vi "Spectrometer Controller.vi"(8 "error in (no error)":errorcluster, 10 "Notifiers":T1, 11 "All Message Queue Cluster":T2) -> (0 "error out":errorcluster)   [LabVIEW 2017]
uses:
  Lib QMH/AllMessageQueue Cluster.ctl
  Lib QMH/Message Cluster.ctl
  Lib Notifier/Notifier.ctl
  Lib Log/Logging.lvlib
  Lib QMH/MessageQueues.lvlib
  Lib Notifier/Notifier.lvlib
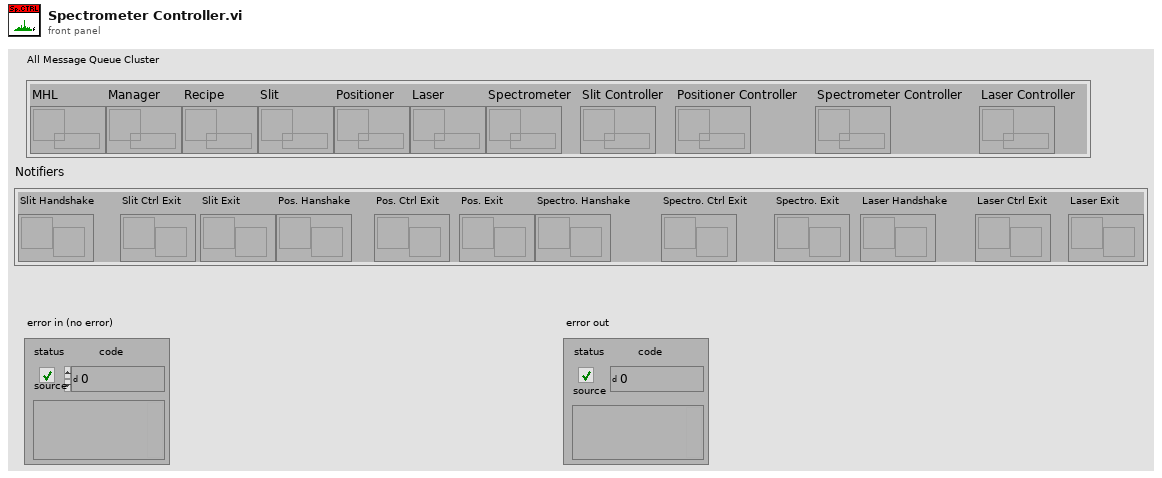
[diagram p1: front panel]
types:
  T1 = typedef "Notifier.lvlib/Notifier.ctl" = cluster{"Slit Handshake":refnum<notifier>, "Slit Ctrl Exit":refnum<notifier>, "Slit Exit":refnum<notifier>, "Pos. Hanshake":refnum<notifier>, "Pos. Ctrl Exit":refnum<notifier>, "Pos. Exit":refnum<notifier>, "Spectro. Hanshake":refnum<notifier>, "Spectro. Ctrl Exit":refnum<notifier>, "Spectro. Exit":refnum<notifier>, "Laser Handshake":refnum<notifier>, "Laser Ctrl Exit":refnum<notifier>, "Laser Exit":refnum<notifier>}
  T2 = typedef "MessageQueues.lvlib/AllMessageQueue Cluster.ctl" = cluster{"MHL":refnum<queue>, "Manager":refnum<queue>, "Recipe":refnum<queue>, "Slit":refnum<queue>, "Positioner":refnum<queue>, "Laser":refnum<queue>, "Spectrometer":refnum<queue>, "Slit Controller":refnum<queue>, "Positioner Controller":refnum<queue>, "Spectrometer Controller":refnum<queue>, "Laser Controller":refnum<queue>}
  T3 = enum16{"open", "replace", "create", "open or create", "replace or create", "replace or create with confirmation"}
  T4 = cluster{"état":bool, "code":i32, "source":string}
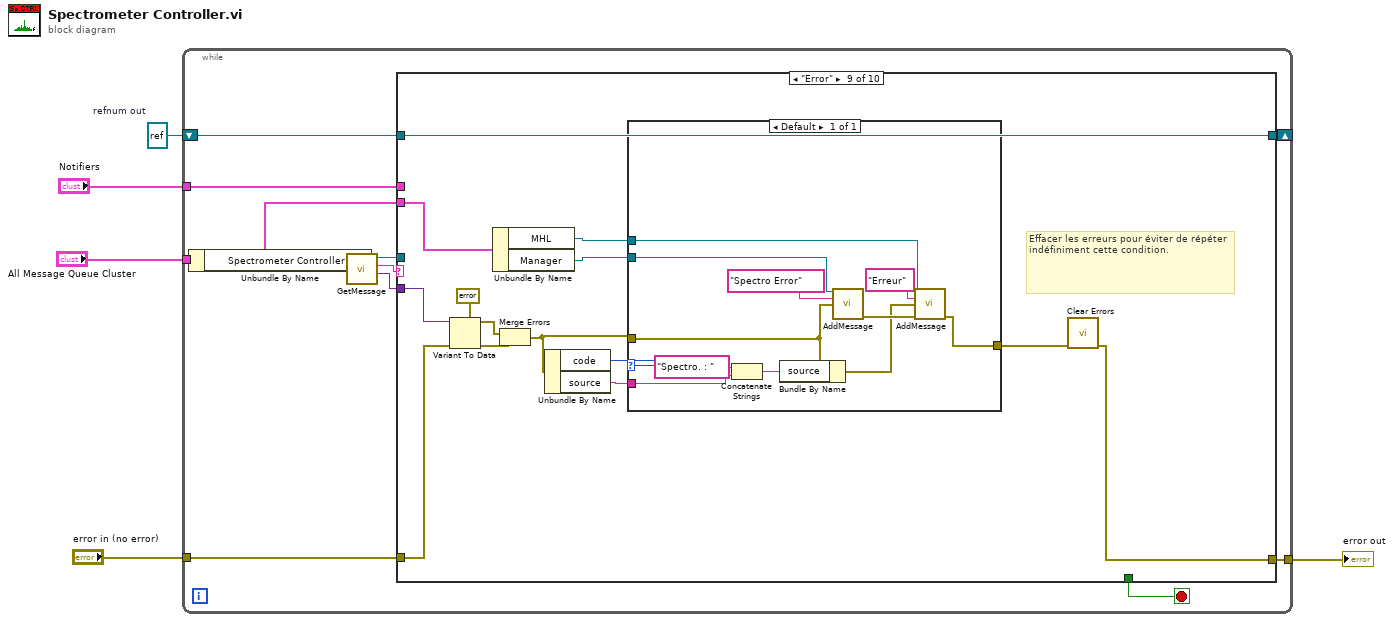
[diagram p0: block diagram]
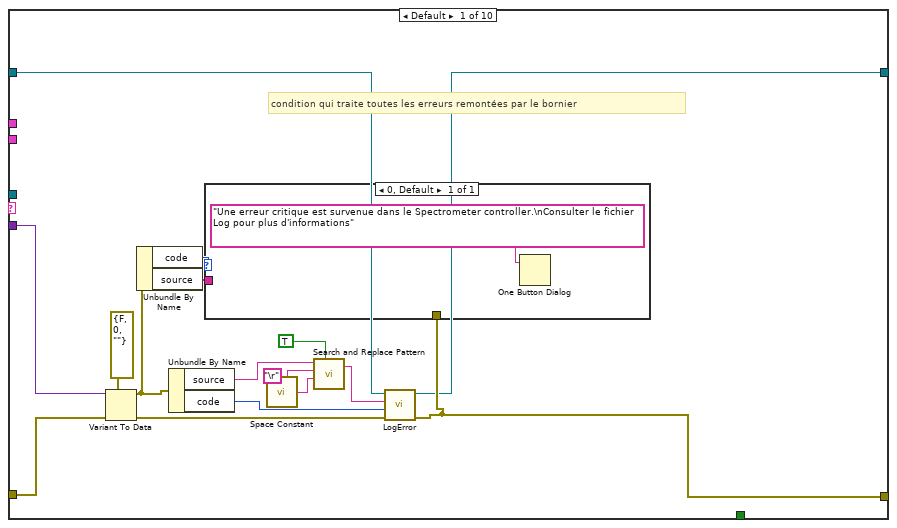
[diagram p2: hidden frame]
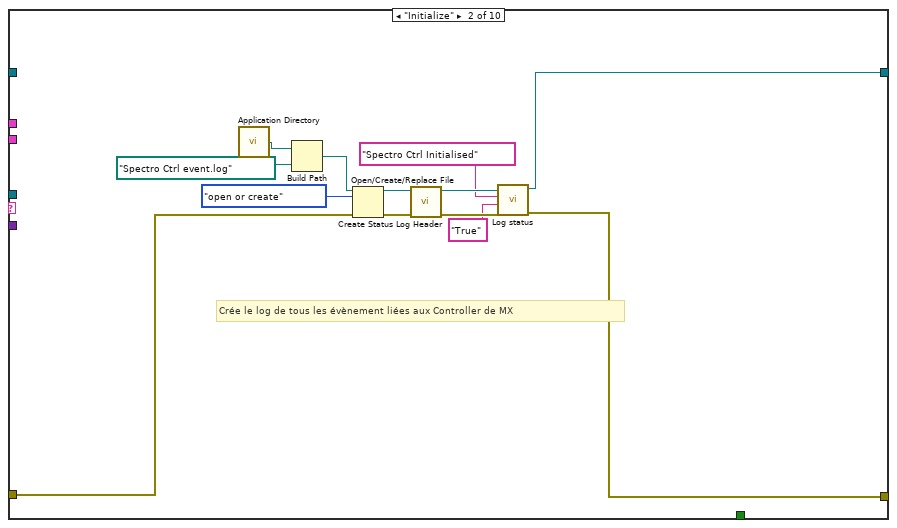
[diagram p3: hidden frame]
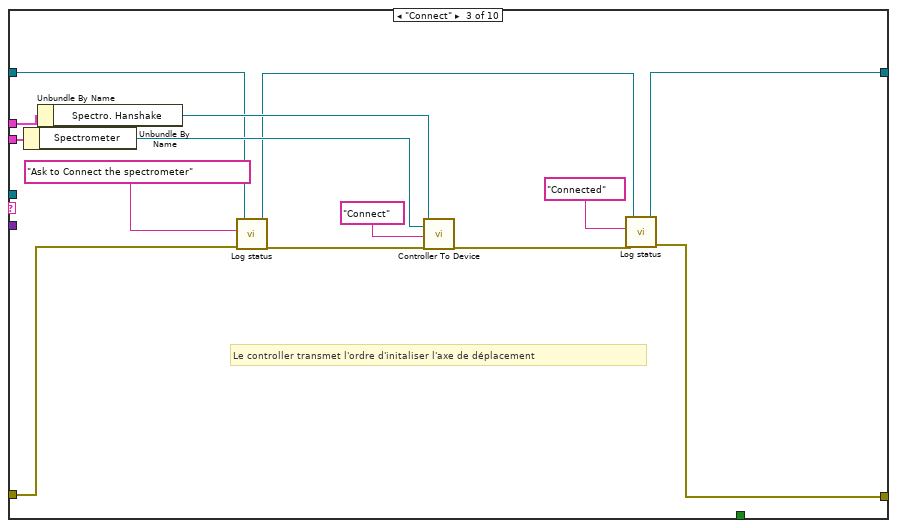
[diagram p4: hidden frame]
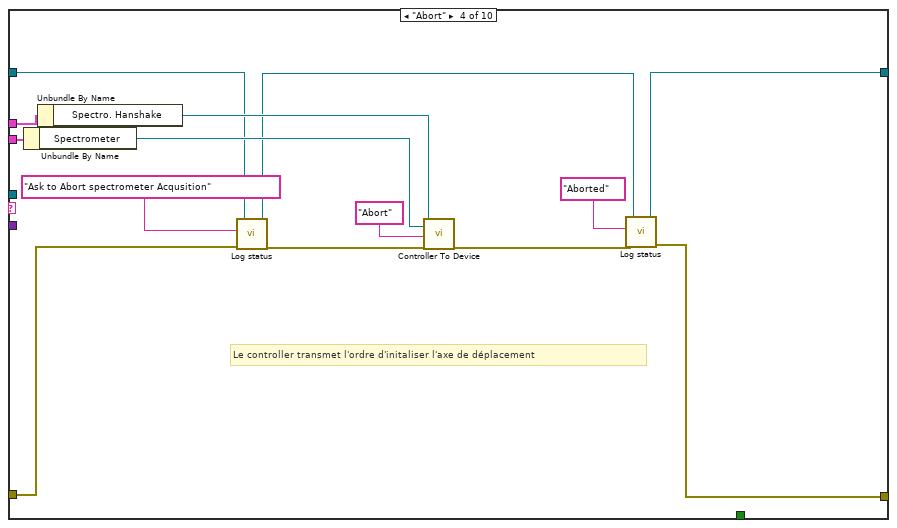
[diagram p5: hidden frame]
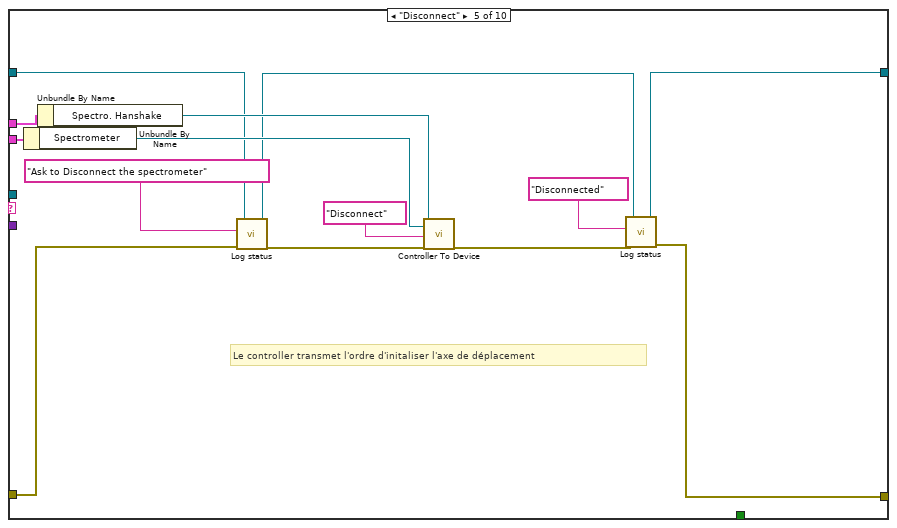
[diagram p6: hidden frame]
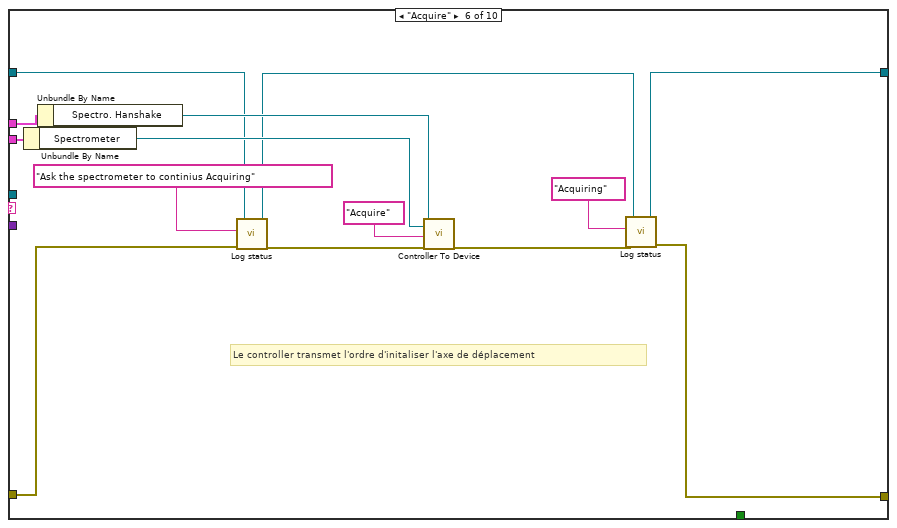
[diagram p7: hidden frame]
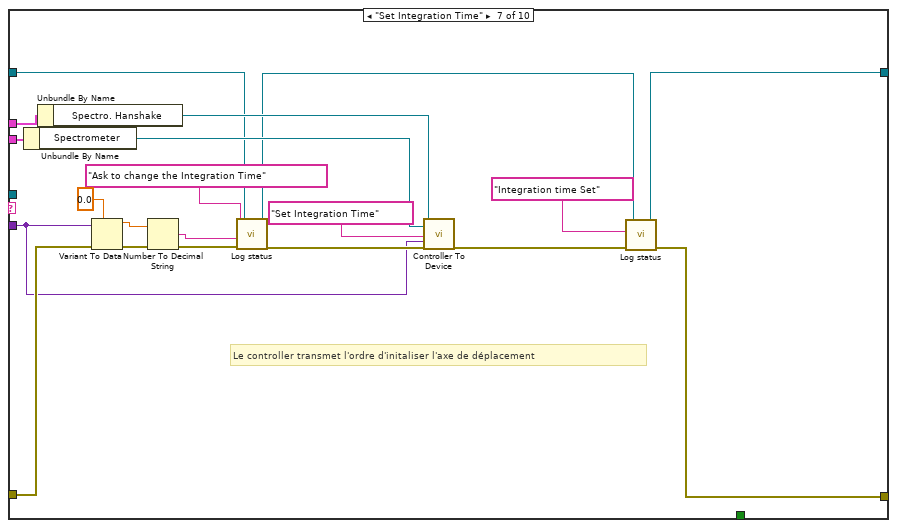
[diagram p8: hidden frame]
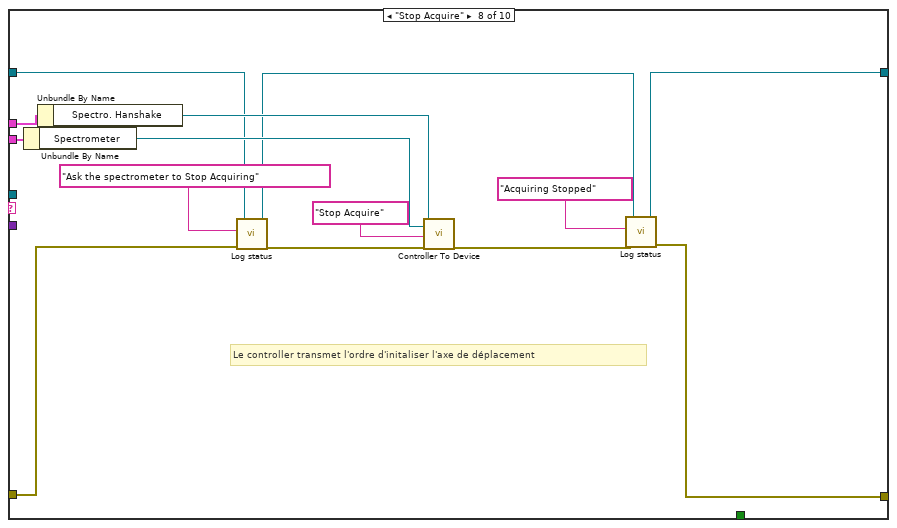
[diagram p9: hidden frame]
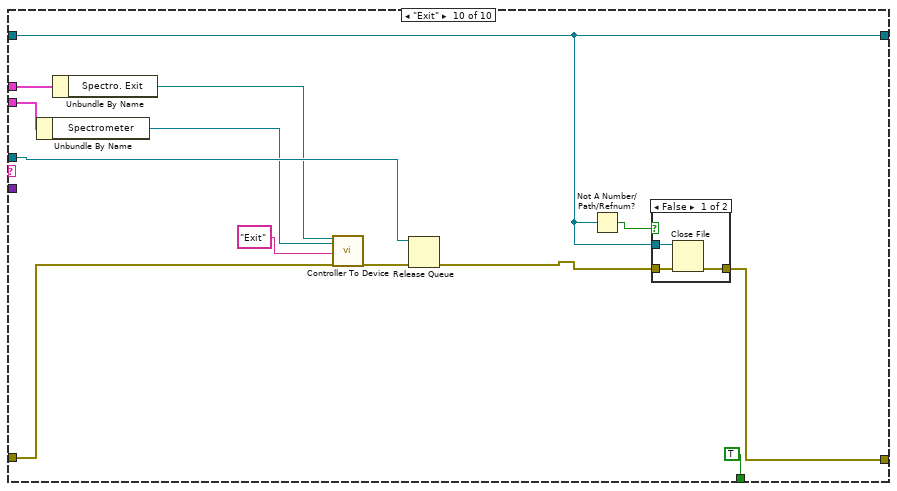
[diagram p10: hidden frame]
diagram:
  w2 = refnum<file> refnum  # refnum out
  n1 = while {
    tunnel: "All Message Queue Cluster" -> [w14]
    tunnel: "Notifiers" -> [w15]
    tunnel: "error in (no error)" -> [w13]
    tunnel: [w6] -> w1
    shift-right: [w8] -> _
    shift-left: w2 -> [w7]
    stop <- w12 stop-if-true
    n2 = Unbundle By Name(w14) -> ("Spectrometer Controller"=w16:refnum<queue>)
    n3 = call "GetMessage.vi"("Message queue"=w16) -> ("Data"=w9:variant, "Message"=w10:string, "Dup Message Queue"=w11:refnum<queue>)  [unwired: 7 in, 1 out]
    n4 = case shown="\"Error\"" w10 {
      tunnel: w15 -> [_ _ w60 w74 w88 w102 w121 w135 _ w170]
      tunnel: w14 -> [_ _ w59 w73 w87 w101 w120 w134 w138 w169]
      tunnel: w13 -> [w21 w36 w48 w62 w76 w90 w108 w123 w140 w165]
      tunnel: [_ _ _ _ _ _ _ _ _ TRUE] -> w12
      tunnel: w11 -> [_ _ _ _ _ _ _ _ _ w171]
      tunnel: w9 -> [w19 _ _ _ _ _ w106 _ w141 _]
      tunnel: [w17 w34 w51 w65 w79 w93 w112 w126 w149 w167] -> w8
      tunnel: w7 -> [w18 _ w55 w69 w83 w97 w116 w130 w149 w167]
      tunnel: [w20 w35 w53 w67 w81 w95 w114 w128 w139 w168] -> w6
      frame Default {
        # "condition qui traite toutes les erreurs remontées par le bornier"
        n5 = Variant To Data(error in=w21, type=errorcluster {"status"=FALSE, "code"=0, "source"=""} ("error in (no error)"), Variant=w19) -> (data=w32:errorcluster, error out=w23:errorcluster)
        n6 = Unbundle By Name(w32) -> ("code"=w30:i32, "source"=w31:string)
        n7 = Unbundle By Name(w32) -> ("source"=w25:string, "code"=w24:i32)
        n8 = call <vilib>:"Space Constant.vi"() -> ("String"=w27:string)
        n9 = call <vilib>:"Search and Replace Pattern.vi"("string"=w25, "regular expression (\"\")"="\r", "replace string (\"\")"=w27, "replace all? (F)"=TRUE) -> ("result string"=w28:string)  [unwired: 1 in, 1 out]
        n10 = call "LogError.vi"("entrée d'erreur"=w23, "Code"=w24, "Source"=w28, "Error log refnum In"=w18) -> ("error out"=w20:errorcluster, "Error log refnum out"=w17:refnum<file>)  [unwired: 6 in]
        n11 = case shown="0, Default" w30 {
          tunnel: w31 -> [_]
          tunnel: w20 -> [_]
          frame 0, Default {
            n12 = One Button Dialog(message="Une erreur critique est survenue dans le Spectrometer controller.\nConsulter le fichier Log pour plus d'informations" ("chaîne de format")) -> ()  [unwired: 1 in, 1 out]
          }
        }
      }
      frame "Initialize" {
        # "Crée le log de tous les évènement liées aux Controller de MX"
        n13 = call <vilib>:"Application Directory.vi"() -> ("Application Directory"=w43:path)
        n14 = Build Path(base path=w43, name or relative path=path "Spectro Ctrl event.log") -> (appended path=w45:path)
        n15 = Open/Create/Replace File(file path (use dialog)=w45, error in=w36, operation (0:open)=T3."open or create" ("opération (0 : open)")) -> (refnum out=w41:refnum<file>, error out=w42:errorcluster)  [unwired: 3 in, 1 out]
        n16 = call "Create Status Log Header.vi"("entrée d'erreur"=w42, "Log File Refnum In"=w41) -> ("sortie d'erreur"=w40:errorcluster, "Log File Refnum out"=w39:refnum<file>)  [unwired: 8 in]
        n17 = call "Log status.vi"("entrée d'erreur"=w40, "Event Data String (-)"="True", "Event string"="Spectro Ctrl Initialised", "Log File Refnum In"=w39) -> ("error out"=w35:errorcluster, "Log File Refnum out"=w34:refnum<file>)  [unwired: 6 in]
      }
      frame "Connect" {
        # "Le controller transmet l'ordre d'initaliser l'axe de déplacement"
        n18 = Unbundle By Name(w59) -> ("Spectrometer"=w57:refnum<queue>)
        n19 = Unbundle By Name(w60) -> ("Spectro. Hanshake"=w58:refnum<notifier>)
        n20 = call "Log status.vi"("entrée d'erreur"=w48, "Event string"="Ask to Connect the spectrometer", "Log File Refnum In"=w55) -> ("error out"=w56:errorcluster, "Log File Refnum out"=w52:refnum<file>)  [unwired: 7 in]
        n21 = call "Controller To Device.vi"("Notifier"=w58, "Message queue"=w57, "Message"="Connect", "entrée d'erreur"=w56) -> ("sortie d'erreur"=w54:errorcluster)  [unwired: 13 in, 2 out]
        n22 = call "Log status.vi"("entrée d'erreur"=w54, "Event string"="Connected", "Log File Refnum In"=w52) -> ("error out"=w53:errorcluster, "Log File Refnum out"=w51:refnum<file>)  [unwired: 7 in]
      }
      frame "Abort" {
        # "Le controller transmet l'ordre d'initaliser l'axe de déplacement"
        n23 = Unbundle By Name(w73) -> ("Spectrometer"=w71:refnum<queue>)
        n24 = Unbundle By Name(w74) -> ("Spectro. Hanshake"=w72:refnum<notifier>)
        n25 = call "Log status.vi"("entrée d'erreur"=w62, "Event string"="Ask to Abort spectrometer Acqusition", "Log File Refnum In"=w69) -> ("error out"=w70:errorcluster, "Log File Refnum out"=w66:refnum<file>)  [unwired: 7 in]
        n26 = call "Controller To Device.vi"("Notifier"=w72, "Message queue"=w71, "Message"="Abort", "entrée d'erreur"=w70) -> ("sortie d'erreur"=w68:errorcluster)  [unwired: 13 in, 2 out]
        n27 = call "Log status.vi"("entrée d'erreur"=w68, "Event string"="Aborted", "Log File Refnum In"=w66) -> ("error out"=w67:errorcluster, "Log File Refnum out"=w65:refnum<file>)  [unwired: 7 in]
      }
      frame "Disconnect" {
        # "Le controller transmet l'ordre d'initaliser l'axe de déplacement"
        n28 = Unbundle By Name(w87) -> ("Spectrometer"=w85:refnum<queue>)
        n29 = Unbundle By Name(w88) -> ("Spectro. Hanshake"=w86:refnum<notifier>)
        n30 = call "Log status.vi"("entrée d'erreur"=w76, "Event string"="Ask to Disconnect the spectrometer", "Log File Refnum In"=w83) -> ("error out"=w84:errorcluster, "Log File Refnum out"=w80:refnum<file>)  [unwired: 7 in]
        n31 = call "Controller To Device.vi"("Notifier"=w86, "Message queue"=w85, "Message"="Disconnect", "entrée d'erreur"=w84) -> ("sortie d'erreur"=w82:errorcluster)  [unwired: 13 in, 2 out]
        n32 = call "Log status.vi"("entrée d'erreur"=w82, "Event string"="Disconnected", "Log File Refnum In"=w80) -> ("error out"=w81:errorcluster, "Log File Refnum out"=w79:refnum<file>)  [unwired: 7 in]
      }
      frame "Acquire" {
        # "Le controller transmet l'ordre d'initaliser l'axe de déplacement"
        n33 = Unbundle By Name(w101) -> ("Spectrometer"=w99:refnum<queue>)
        n34 = Unbundle By Name(w102) -> ("Spectro. Hanshake"=w100:refnum<notifier>)
        n35 = call "Log status.vi"("entrée d'erreur"=w90, "Event string"="Ask the spectrometer to continius Acquiring", "Log File Refnum In"=w97) -> ("error out"=w98:errorcluster, "Log File Refnum out"=w94:refnum<file>)  [unwired: 7 in]
        n36 = call "Controller To Device.vi"("Notifier"=w100, "Message queue"=w99, "Message"="Acquire", "entrée d'erreur"=w98) -> ("sortie d'erreur"=w96:errorcluster)  [unwired: 13 in, 2 out]
        n37 = call "Log status.vi"("entrée d'erreur"=w96, "Event string"="Acquiring", "Log File Refnum In"=w94) -> ("error out"=w95:errorcluster, "Log File Refnum out"=w93:refnum<file>)  [unwired: 7 in]
      }
      frame "Set Integration Time" {
        # "Le controller transmet l'ordre d'initaliser l'axe de déplacement"
        n38 = Unbundle By Name(w120) -> ("Spectrometer"=w118:refnum<queue>)
        n39 = Unbundle By Name(w121) -> ("Spectro. Hanshake"=w119:refnum<notifier>)
        n40 = Variant To Data(error in=w108, type=0.0, Variant=w106) -> (data=w104:dbl, error out=w107:errorcluster)
        n41 = Number To Decimal String(number=w104) -> (decimal integer string=w103:string)  [unwired: 1 in]
        n42 = call "Log status.vi"("entrée d'erreur"=w107, "Event Data String (-)"=w103, "Event string"="Ask to change the Integration Time", "Log File Refnum In"=w116) -> ("error out"=w117:errorcluster, "Log File Refnum out"=w113:refnum<file>)  [unwired: 6 in]
        n43 = call "Controller To Device.vi"("Notifier"=w119, "Message queue"=w118, "Message"="Set Integration Time", "Data"=w106, "entrée d'erreur"=w117) -> ("sortie d'erreur"=w115:errorcluster)  [unwired: 12 in, 2 out]
        n44 = call "Log status.vi"("entrée d'erreur"=w115, "Event string"="Integration time Set", "Log File Refnum In"=w113) -> ("error out"=w114:errorcluster, "Log File Refnum out"=w112:refnum<file>)  [unwired: 7 in]
      }
      frame "Stop Acquire" {
        # "Le controller transmet l'ordre d'initaliser l'axe de déplacement"
        n45 = Unbundle By Name(w134) -> ("Spectrometer"=w132:refnum<queue>)
        n46 = Unbundle By Name(w135) -> ("Spectro. Hanshake"=w133:refnum<notifier>)
        n47 = call "Log status.vi"("entrée d'erreur"=w123, "Event string"="Ask the spectrometer to Stop Acquiring", "Log File Refnum In"=w130) -> ("error out"=w131:errorcluster, "Log File Refnum out"=w127:refnum<file>)  [unwired: 7 in]
        n48 = call "Controller To Device.vi"("Notifier"=w133, "Message queue"=w132, "Message"="Stop Acquire", "entrée d'erreur"=w131) -> ("sortie d'erreur"=w129:errorcluster)  [unwired: 13 in, 2 out]
        n49 = call "Log status.vi"("entrée d'erreur"=w129, "Event string"="Acquiring Stopped", "Log File Refnum In"=w127) -> ("error out"=w128:errorcluster, "Log File Refnum out"=w126:refnum<file>)  [unwired: 7 in]
      }
      frame "Error" {
        # "Effacer les erreurs pour éviter de répéter indéfiniment cette condition."
        n50 = Variant To Data(error in=w140, type=T4 {"état"=FALSE, "code"=0, "source"=""} ("sortie d'erreur"), Variant=w141) -> (data=w146:T4, error out=w147:errorcluster)
        n51 = Unbundle By Name(w138) -> ("MHL"=w137:refnum<queue>, "Manager"=w142:refnum<queue>)
        n52 = Merge Errors(w146, w147) -> (w143:errorcluster)
        n53 = Unbundle By Name(w143) -> ("code"=w144:i32, "source"=w136:string)
        n54 = case shown="Default" w144 {
          tunnel: [w157] -> w145
          tunnel: w143 -> [w154]
          tunnel: w142 -> [w155]
          tunnel: w137 -> [w156]
          tunnel: w136 -> [w152]
          frame Default {
            n55 = Concatenate Strings("Spectro. : " ("string"), w152) -> (w151:string)
            n56 = Bundle By Name(cluster=w154, "source"=w151) -> (w150:errorcluster)
            n57 = call "AddMessage.vi"("Message queue"=w155, "Message"="Spectro Error", "Data"=w154) -> ("error out"=w158:errorcluster)  [unwired: 11 in, 1 out]
            n58 = call "AddMessage.vi"("Message queue"=w156, "Message"="Erreur", "Data"=w150, "entrée d'erreur (pas d'erreur)"=w158) -> ("error out"=w157:errorcluster)  [unwired: 10 in, 1 out]
          }
        }
        n59 = call <vilib>:"Clear Errors.vi"("error in (no error)"=w145) -> ("error out"=w139:errorcluster)  [unwired: 5 in, 1 out]
      }
      frame "Exit" {
        n60 = Unbundle By Name(w169) -> ("Spectrometer"=w162:refnum<queue>)
        n61 = Unbundle By Name(w170) -> ("Spectro. Exit"=w163:refnum<notifier>)
        n62 = call "Controller To Device.vi"("Notifier"=w163, "Message queue"=w162, "Message"="Exit", "entrée d'erreur"=w165) -> ("sortie d'erreur"=w166:errorcluster)  [unwired: 13 in, 2 out]
        n63 = Release Queue(queue=w171, error in (no error)=w166) -> (error out=w161:errorcluster)  [unwired: 1 in, 2 out]
        n64 = Not A Number/Path/Refnum?(number/path/refnum=w167) -> (NaN/Path/Refnum?=w172:bool)
        n65 = case shown="False" w172 {
          tunnel: [w176 w177] -> w168
          tunnel: w161 -> [w175 w177]
          tunnel: w167 -> [w174 _]
          frame False {
            n66 = Close File(refnum=w174, error in=w175) -> (error out=w176:errorcluster)  [unwired: 1 out]
          }
          frame True {
          }
        }
      }
    }
  }
  "error out" <- w1
